vi "prezzo treno.vi"() -> ()   [LabVIEW 2013]
panel:
  in  "invalido":bool
  out "prezzo":dbl
  in  "classe":bool
  in  "treno":string(combo)
  in  "entra":bool
  in  "età":dbl
  in  "distanza":dbl
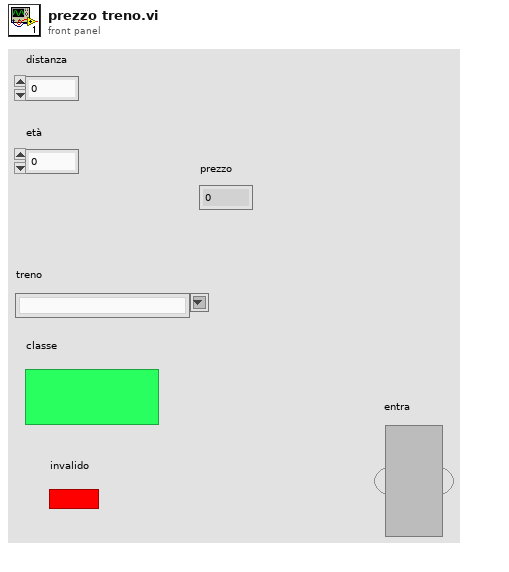
[diagram p1: front panel]
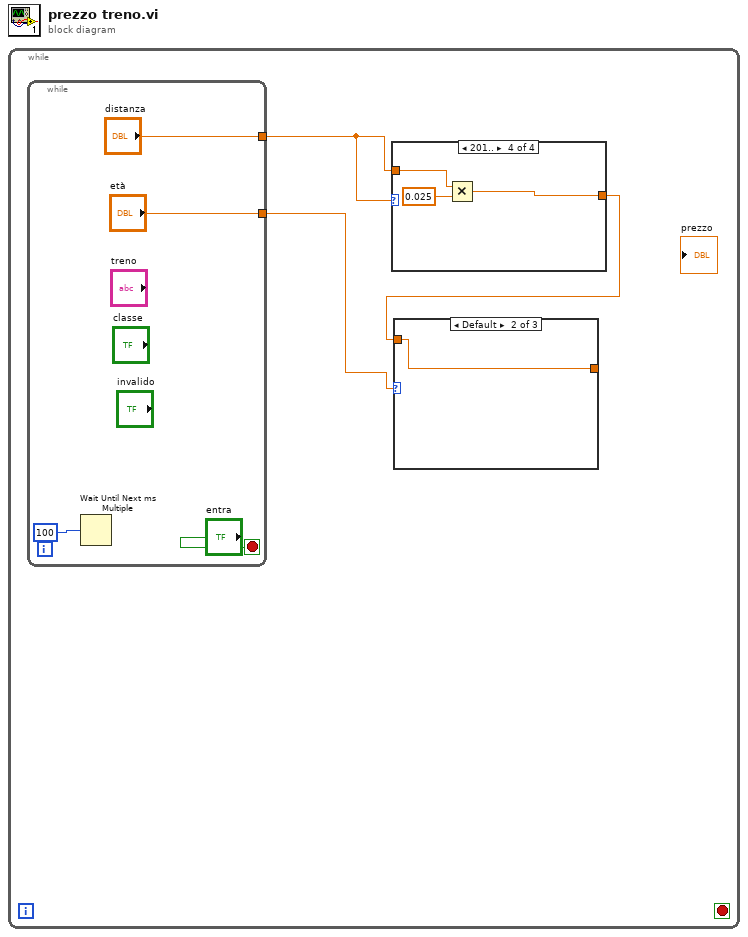
[diagram p0: block diagram]
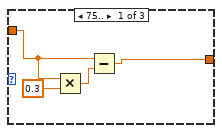
[diagram p2: hidden frame]
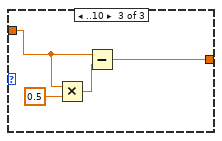
[diagram p3: hidden frame]
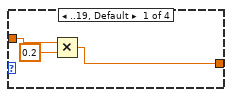
[diagram p4: hidden frame]
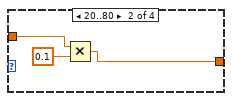
[diagram p5: hidden frame]
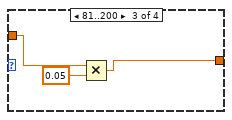
[diagram p6: hidden frame]
diagram:
  n1 = while {
    stop <- _ stop-if-true
    n2 = while {
      tunnel: ["distanza"] -> w2
      tunnel: ["età"] -> w1
      stop <- "entra" stop-if-true
      n3 = Wait Until Next ms Multiple(millisecond multiple=u32 100) -> ()  [unwired: 1 out]
    }
    n4 = case shown="201.." w2 {
      tunnel: w2 -> [w15 w18 w21 w24]
      tunnel: [w13 w16 w19 w22] -> w3
      frame ..19, Default {
        n5 = Multiply(x=w15, y=0.2) -> (x*y=w13:dbl)
      }
      frame 20..80 {
        n6 = Multiply(x=w18, y=0.1) -> (x*y=w16:dbl)
      }
      frame 81..200 {
        n7 = Multiply(x=w21, y=0.05) -> (x*y=w19:dbl)
      }
      frame 201.. {
        n8 = Multiply(x=w24, y=0.025) -> (x*y=w22:dbl)
      }
    }
    n9 = case shown="Default" w1 {
      tunnel: w3 -> [w7 w8 w12]
      tunnel: [w4 w8 w9] -> _
      frame 75.. {
        n10 = Multiply(x=w7, y=0.3) -> (x*y=w5:dbl)
        n11 = Subtract(x=w7, y=w5) -> (x-y=w4:dbl)
      }
      frame Default {
      }
      frame ..10 {
        n12 = Multiply(x=w12, y=0.5) -> (x*y=w10:dbl)
        n13 = Subtract(x=w12, y=w10) -> (x-y=w9:dbl)
      }
    }
  }
